vi "Add I32 to HashTable.vi"(8 "error in (no error)":errorcluster caption="错误输入（无错误）", 9 "Value":i32, 10 "Name":string, 11 "Contstant Base 输入":refnum<class "Tag Data.lvclass"> caption="DNL_LabVIEW Object in") -> (0 "error out":errorcluster caption="错误输出", 3 "Contstant Base 输出":refnum<class "Tag Data.lvclass"> caption="DNL_LabVIEW Object out")   [LabVIEW 2013, in "Tag Data.lvclass"]
uses:
  Tag Data.lvclass
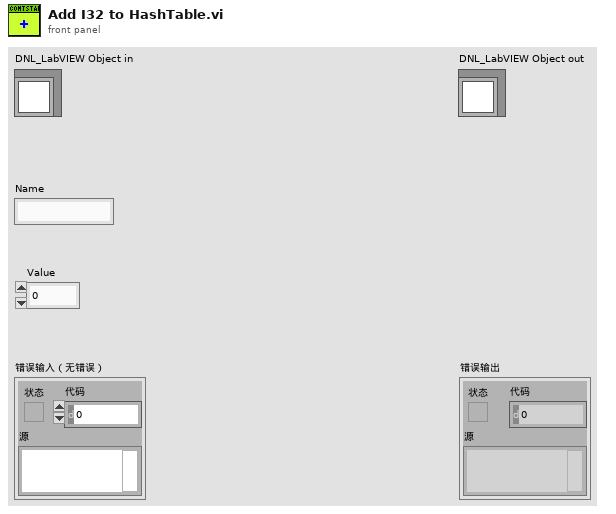
[diagram p1: front panel]
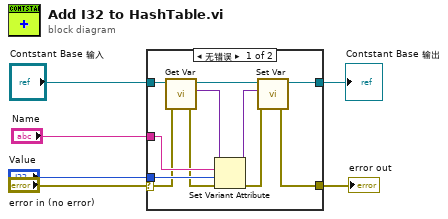
[diagram p0: block diagram]
diagram:
  n1 = case shown="无错误" "error in (no error)" {
    selector: "error in (no error)" -> [w10 w19]
    tunnel: [w7 w19] -> w5
    tunnel: [w13 w18] -> w3
    tunnel: "Contstant Base 输入" -> [w17 w18]
    tunnel: "Name" -> [w12 _]
    tunnel: "Value" -> [w11 _]
    frame No Error {
      n2 = call-dynamic "Get Var.vi"("error in (no error)"=w10, "Contstant Base输入"=w17) -> ("error out"=w9:errorcluster, "Var"=w16:variant, "Contstant Base输出"=w14:refnum<class "Tag Data.lvclass">)  [unwired: 7 in]
      n3 = Set Variant Attribute(Variant=w16, name=w12, value=w11, error in=w9) -> (Variant out=w15:variant, error out=w8:errorcluster)  [unwired: 1 out]
      n4 = call-dynamic "Set Var.vi"("error in (no error)"=w8, "Var"=w15, "Contstant Base输入"=w14) -> ("error out"=w7:errorcluster, "Contstant Base输出"=w13:refnum<class "Tag Data.lvclass">)  [unwired: 7 in]
    }
    frame Error {
    }
  }
  "error out" <- w5
  "Contstant Base 输出" <- w3
